vi "writeToXML.vi"(8 "error in (no error)":errorcluster, 11 "IAA in":refnum<class "IAA.lvclass">) -> (0 "error out":errorcluster, 2 "XML out":string, 3 "IAA out":refnum<class "IAA.lvclass">)   [LabVIEW 2009, in "IAA.lvclass"]
uses:
  IAA.lvclass
  Common/UnitsAndXML/FlattenItemWithUnitToXML/FlattenPlaneAngleToXML/PlaneAngleUnit.ctl
  IAA.lvclass/IAA.ctl
  Common/UnitsAndXML/FlattenItemWithUnitToXML/FlattenPlaneAngleToXML/typeMethods/flattenPlaneAngleToXML_Scalar.vi
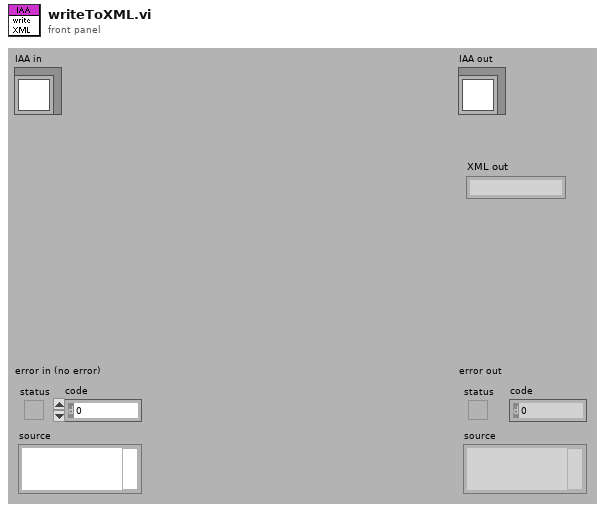
[diagram p1: front panel]
types:
  T1 = typedef "PlaneAngleUnit.ctl" = enum16{"rad", "deg", "'", "\""}
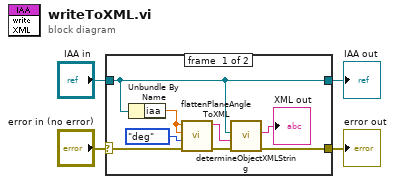
[diagram p0: block diagram]
diagram:
  n1 = case shown="No Error" "error in (no error)" {
    selector: "error in (no error)" -> [w10 w14]
    tunnel: [w6 w14] -> w3
    tunnel: [w9 w13] -> w1
    tunnel: "IAA in" -> [w9 w13]
    frame #0 {
      n2 = Unbundle By Name(w9) -> ("iaa"=w12:dbl[unit])
      n3 = call-poly "flattenPlaneAngleToXML.vi"("error in (no error)"=w10, "planeAngleUnitInXML"=PlaneAngleUnit."deg", "planeAngleAgain"=w12, "planeAngle"=w12) -> ("error out"=w7:errorcluster, "xmlString"=w8:string)  [unwired: 6 in]
      n4 = call "determineObjectXMLString.vi"("error in (no error)"=w7, "classContentsString"=w8, "LabVIEW Object"=w9) -> ("error out"=w6:errorcluster, "outputXMLString"=→"XML out":string)  [unwired: 7 in]
    }
    frame #1 {
    }
  }
  "error out" <- w3
  "IAA out" <- w1
